vi "USB_Locate.vi"(8 "error in (no error)":errorcluster, 9 "pid":u16=2048 format="%x", 10 "vid":u16=2048 format="%04x") -> (0 "error out":errorcluster, 2 "found?":bool, 3 "VISA Resource Name":refnum<visa-resource-name>)   [LabVIEW 2010, in "lib1299.lvlib"]
uses:
  lib1299.lvlib
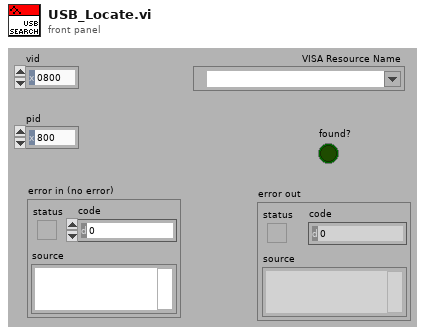
[diagram p1: front panel]
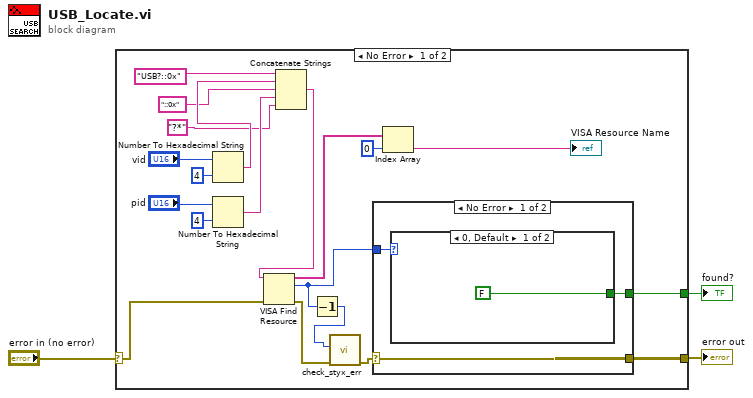
[diagram p0: block diagram]
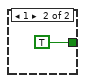
[diagram p2: hidden frame]
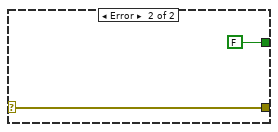
[diagram p3: hidden frame]
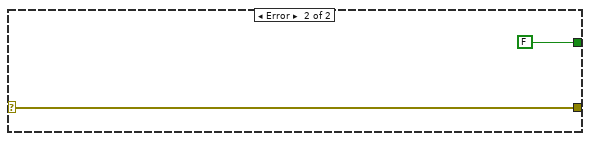
[diagram p4: hidden frame]
diagram:
  n1 = case shown="No Error" "error in (no error)" {
    selector: "error in (no error)" -> [w11 w32]
    tunnel: [w22 w32] -> w3
    tunnel: [w23 FALSE ("found?")] -> w1
    frame No Error {
      n2 = Number To Hexadecimal String(1:i16 4 ("width (-)"), 2:"vid") -> (0:w18:string)
      n3 = Number To Hexadecimal String(1:i16 4 ("width (-)"), 2:"pid") -> (0:w14:string)
      n4 = Concatenate Strings("USB?::0x", w18, "::0x", w14, "?*") -> (w12:string)
      n5 = VISA Find Resource(8:w11, 11:w12) -> (0:w5:errorcluster, 2:w7:u32, 3:w9:string[])  [unwired: 1 out]
      n6 = Decrement(x=w7) -> (x-1=w6:u32)
      n7 = call "check_styx_err.vi"("error in (no error)"=w5, "return val"=w6) -> ("error out"=w4:errorcluster)  [unwired: 9 in]
      n8 = case shown="No Error" w4 {
        selector: w4 -> [w24 w29]
        tunnel: [w26 FALSE ("found?")] -> w23
        tunnel: [w24 w29] -> w22
        tunnel: w7 -> [w25 _]
        frame No Error {
          n9 = case shown="0, Default" w25 {
            tunnel: [FALSE ("found?") TRUE ("found?")] -> w26
            frame 0, Default {
            }
            frame 1 {
            }
          }
        }
        frame Error {
        }
      }
      n10 = Index Array(array=w9, index=0) -> (element=→"VISA Resource Name":string)
    }
    frame Error {
    }
  }
  "error out" <- w3
  "found?" <- w1
